vi "table_get_subtable_keys.vi"(7 "subtables":string[](array[string]), 8 "error in (no error)":errorcluster, 11 "Table in":refnum<class "Table.lvclass">) -> (0 "error out":errorcluster, 1 "keys":string[](array[string]), 2 "found subtable?":bool, 3 "Table out":refnum<class "Table.lvclass">)   [LabVIEW 2020, in "toml.lvclass"]
uses:
  Table/Table.lvclass
  toml.lvclass
  toml.lvclass/toml.ctl
  Item/Item.lvclass
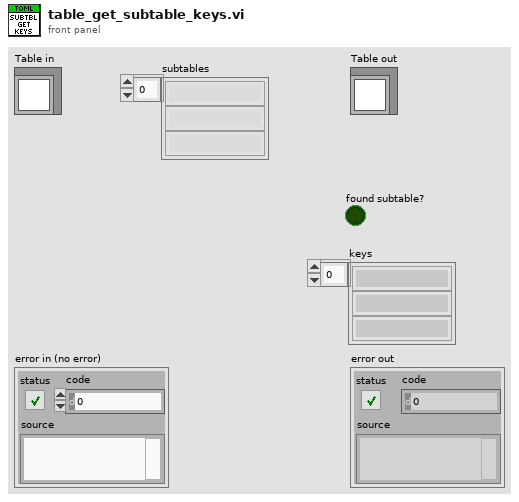
[diagram p1: front panel]
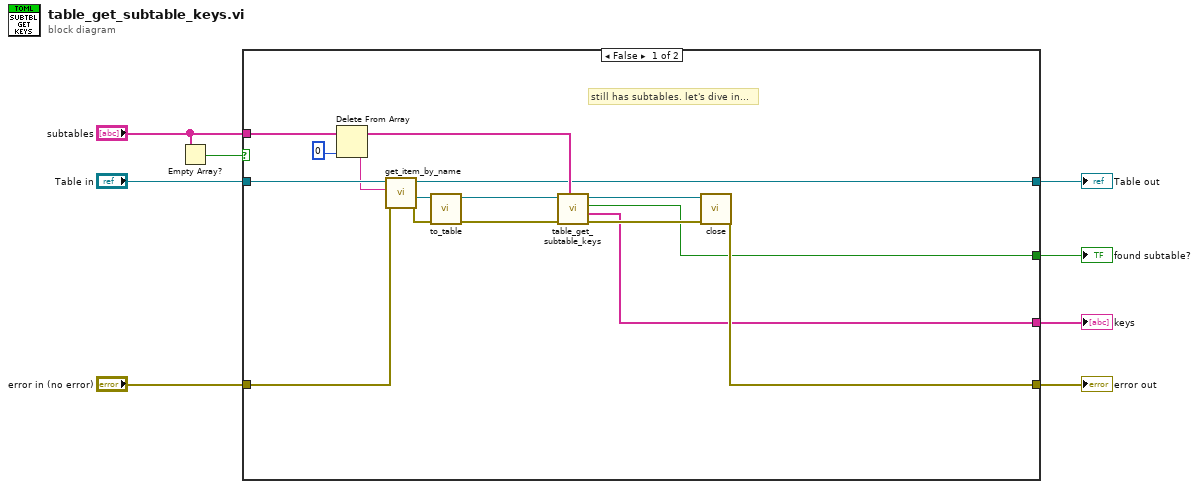
[diagram p0: block diagram]
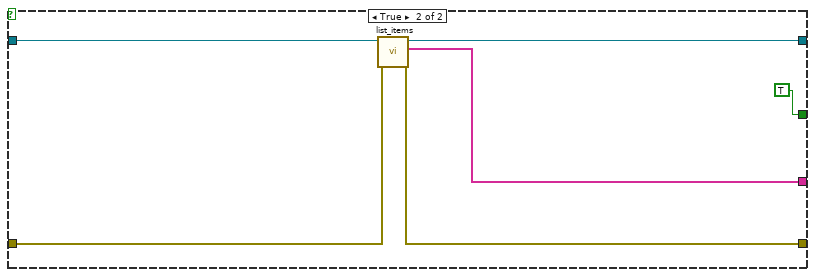
[diagram p2: hidden frame]
diagram:
  n1 = Empty Array?(array="subtables") -> (empty?=w4:bool)
  n2 = case shown="False" w4 {
    tunnel: [w13 w26] -> w8
    tunnel: [w18 w29] -> w7
    tunnel: "Table in" -> [w21 w30]
    tunnel: "error in (no error)" -> [w20 w25]
    tunnel: "subtables" -> [w24 _]
    tunnel: [w12 w28] -> w2
    tunnel: [w9 TRUE ("found subtable?")] -> w1
    frame False {
      # "still has subtables. let's dive in..."
      n3 = Delete From Array(array=w24, index=0) -> (deleted portion=w16:string, array with subset deleted=w22:string[])  [unwired: 1 in]
      n4 = call "get_item_by_name.vi"("error in (no error)"=w20, "item_name"=w16, "Table in"=w21) -> ("error out"=w17:errorcluster, "Item"=w19:refnum<class "Item.lvclass">, "Table out"=w18:refnum<class "Table.lvclass">)  [unwired: 6 in]
      n5 = call "to_table.vi"("error in (no error)"=w17, "Item in"=w19) -> ("error out"=w11:errorcluster, "Table"=w10:refnum<class "Table.lvclass">)  [unwired: 8 in]
      n6 = call "table_get_subtable_keys.vi"("subtables"=w22, "error in (no error)"=w11, "Table in"=w10) -> ("error out"=w14:errorcluster, "keys"=w12:string[], "found subtable?"=w9:bool, "Table out"=w15:refnum<class "Table.lvclass">)  [unwired: 5 in]
      n7 = call "close.vi"("error in (no error)"=w14, "Table in"=w15) -> ("error out"=w13:errorcluster)  [unwired: 9 in]
    }
    frame True {
      n8 = call "list_items.vi"("error in (no error)"=w25, "Table in"=w30) -> ("error out"=w26:errorcluster, "items"=w28:string[], "Table out"=w29:refnum<class "Table.lvclass">)  [unwired: 7 in]
    }
  }
  "error out" <- w8
  "keys" <- w2
  "Table out" <- w7
  "found subtable?" <- w1
